vi "Dashboard Main.vi"() -> ()   [LabVIEW 2014]
uses:
  <vilib>/event_ctls.llb/eventvkey.ctl
  <vilib>/Rock Robotics/WPI/Dashboard/WPI_DashboardLogging Global.vi
  <vilib>/Rock Robotics/Network Tables/SD Read Number.vi
  <vilib>/Rock Robotics/Network Tables/SD Read Boolean.vi
  <vilib>/Utility/config.llb/Write Key (String).vi
  <vilib>/Utility/config.llb/Write Key (I32).vi
  <vilib>/Utility/config.llb/NI_LVConfig.lvlib
panel:
  out "Camera Active":bool
  out "Image Message":string="Timeout in Camera Communications"
  out "Camera Image":T1(plugin-control)
  in  "TCP":refnum<k5>
  in  "Rec Mode":enum32{"Stop", "Record", "Playback"}(radio)
  in  "Vision":u16(ring) items=["Camera Off", "USB Camera SW", "USB Camera HW", "IP Camera"]
  in  "Dashboard Tab":T2(tab)
  in  "Camera Settings":T3={"Frame Rate"=30, "Compression"=30, "Size"=1} {"Frame Rate" scale=1.0..30.0; "Size" items=["640x480", "320x240", "160x120"]}
  out "MotorChart R":cluster{"Numeric":dbl, "Numeric":dbl}(graph)
  out "MotorChart L":T4(graph)
  out "MotorSliders R":cluster{"MotorSlide1":dbl, "MotorSlide2":dbl} {"MotorSlide2" scale=-1.0..1.0 scale format="%#_2e"; "MotorSlide1" scale=-1.0..1.0 scale format="%#_2e"}
  out "MotorSliders L":T5 {"MotorSlide4 2" scale=0.0..14.0 scale format="%#_2e"; "MotorSlide2" scale=-1.0..1.0 scale format="%#_2e"; "MotorSlide1" scale=-1.0..1.0 scale format="%#_2e"}
  out "Gyro":dbl(knob) scale=0.0..360.0
  out "JS1 Z":dbl(slide) scale=-1.0..1.0 scale format="%#_2e"
  out "JS1 Graph":cluster{"X":dbl, "Y":dbl}[](graph)
  out "JS1 Buttons":T6
  out "JS2 Z":dbl(slide) scale=-1.0..1.0 scale format="%#_2e"
  out "JS2 Graph":cluster{"X":dbl, "Y":dbl}[](graph)
  out "JS2 Buttons":T6
  out "Mode":T7(ring)=enum."Auto Disabled"
  in  "DB Camera Config":bool
  out "fps":dbl format="%#.1g"
  out "Mbps":dbl format="%#.1g"
  out "Mbps 2":bool
  out "Accel Y":dbl
  out "Accel Z":dbl
  out "Accel X":dbl
  out "LimitSW1":bool
  out "Camera IP":string
  in  "DB/String 9":string
  in  "DB/String 8":string
  in  "DB/String 7":string
  in  "DB/String 6":string
  in  "DB/String 5":string
  in  "DB/String 4":string
  in  "DB/String 3":string
  in  "DB/String 2":string
  in  "DB/String 1":string
  in  "DB/String 0":string
  in  "DB/Slider 0":dbl(slide) scale=0.0..5.0
  in  "DB/Slider 1":dbl(slide) scale=0.0..5.0
  in  "DB/Slider 2":dbl(slide) scale=0.0..5.0
  in  "DB/Slider 3":dbl(slide) scale=0.0..5.0
  out "DB/LED 3":bool
  out "DB/LED 2":bool
  out "DB/LED 1":bool
  out "DB/LED 0":bool
  in  "DB/Button 3":bool
  in  "DB/Button 2":bool
  in  "DB/Button 1":bool
  in  "DB/Button 0":bool caption="New Name"
  in  "Test Slider":dbl(slide) scale=0.0..100.0 scale format="%#_3g"
  in  "On/Off":bool caption="Solenoid"
  in  "Test Name":u16(ring) items=["Select the test to run...", "Example Test", "-------------------------------", "List of tests is built in robot code.", "Replace with your own automated tests."]
  in  "Test Tree":string(tree)
  in  "Motor":cluster{"Value":dbl, "Enable":bool} {"Value" scale=-1.0..1.0 scale format="%#_3g"}
  out "Progress":T8 {"Test Progress" scale=0.0..100.0}
  in  "Rev/Fwd":cluster{"Forward":bool, "Reverse":bool}
  in  "Test Ring":u16(ring) items=["Monochrome", "Color"]
  in  "Listbox":i32(listbox)
  out "Tree":string(tree)
  out "Boolean":bool
  # "Left"
  # "Front"
  # "Right"
  # "Battery"
  # "This tab is a great place for autonomous settings and robot-specific values.\nPlace controls and indicators inside this tab and match name to\nDashboard Variables on robot. You can also delete this comment."
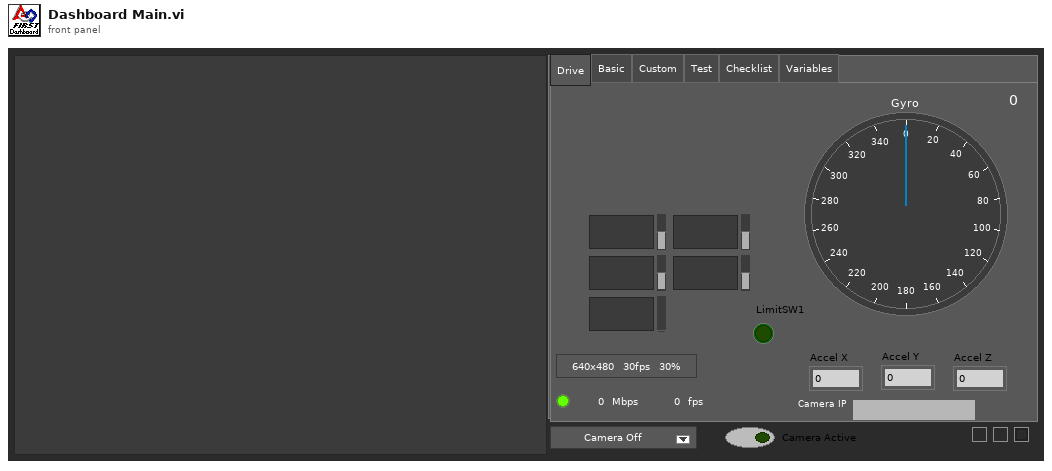
[diagram p1: front panel]
types:
  T1 = typedef "IMAQ Image.ctl" = refnum<image>
  T2 = enum32{"Drive", "Basic", "Custom", "Test", "Checklist", "Variables"}
  T3 = cluster{"Frame Rate":i32, "Compression":i32, "Size":u16}
  T4 = cluster{"Numeric":dbl, "Numeric":dbl, "Battery V":dbl}
  T5 = cluster{"MotorSlide1":dbl, "MotorSlide2":dbl, "MotorSlide4 2":dbl}
  T6 = cluster{bool, bool, bool, bool, bool, bool, bool, bool, bool, bool, bool, bool}
  T7 = enum8{"Tele-Op Disabled", "Tele-Op Enabled", "Auto Disabled", "Auto Enabled", "Test Disabled", "Test Enabled", "Disconnected", "No Code", "E-Stop"}
  T8 = cluster{"Test Progress":u8, "Test Progress Text":string}
  T9 = typedef "Image Type" = u32
  T10 = cluster{"Camera Image":refnum<vi>, "Dashboard Tab":refnum<vi>, "Boolean":refnum<vi>, "Vision":refnum<vi>, "Rec Mode":refnum<vi>, "Test Slider":refnum<vi>, "On/Off ":refnum<vi>, "Test Ring":refnum<vi>, "Rev/Fwd":refnum<vi>, "Test Name":refnum<vi>, "Motor":refnum<vi>, "Progress":refnum<vi>, "CheckList":refnum<vi>, "Tree":refnum<vi>, "Test Tree":refnum<vi>}
  T11 = cluster{"Error Strings":string, "Disable Counts":cluster{u16, u16}, "Rail Faults":cluster{u16, u16, u16}, "Robot IP":string, "DB Mode":u8, "Event Info":cluster{"Name":string, "Type":u8, "Number":u16, "Replay":u8}, "Camera Addr":string}
  T12 = cluster{"Storage":cluster{"Disk Free":u64, "RAM Block":u32, "RAM free":u32}, "CPU Utilization":cluster{"CPU % ISR":sgl, "CPU % Time Crit":sgl, "CPU % Timed Str":sgl, "CPU % High":sgl, "CPU % Above":sgl, "CPU % Normal":sgl, "CPU % Low":sgl}, "CAN":cluster{"% Bus Utilization":sgl, "Bus Off Cnt":u32, "TX_FIFO Full Cnt":u32, "Receive Error Cnt":u8, "Transmit Error Cnt":u8}, "HID":cluster{"HID Outputs":u32, "Rumble Low":u16, "Rumble High":u16}[]}
  T13 = cluster{"Status bits":cluster{"Test Mode":bool, "Autonomous":bool, "Enabled":bool, "Code Start":bool, "Brownout":bool, "Reserved 2":bool, "Reserved 3":bool, "E-Stop":bool}, "Code Trace":cluster{"Disabled":bool, "TeleOp":bool, "Auto":bool, "Test":bool}, "Controller Type":enum16{"unknown", "cRIO", "roboRio"}, "Code?":enum16{"unknown", "noCode", "code"}, "Battery V":dbl}
  T14 = cluster{"Control Bits":cluster{"TestMode":bool, "Autonomous":bool, "Enabled":bool, "FMS Present":bool, bool, bool, bool, "E-Stop":bool}, "Team Station ":u8, "Countdown":sgl, "Joystick Values":cluster{"Axes":dbl[], "Buttons":bool[], "POVs":i16[]}[]}
  T15 = cluster{"Axes":dbl[], "Buttons":bool[], "POVs":i16[]}[]
  T16 = cluster{"Axes":dbl[], "Buttons":bool[], "POVs":i16[]}
  T17 = cluster{"Buttons[0]":bool, "Buttons[1]":bool, "Buttons[2]":bool, "Buttons[3]":bool, "Buttons[4]":bool, "Buttons[5]":bool, "Buttons[6]":bool, "Buttons[7]":bool, "Buttons[8]":bool, "Buttons[9]":bool, "Buttons[10]":bool, "Buttons[11]":bool}
  T18 = typedef "NI_LVConfig.lvlib/Config Data RefNum.ctl" = refnum<k1>
  T19 = cluster{"Operation":enum16{"Update", "Clear"}, "Color Box":u32}[]
  T20 = typedef "eventvkey.ctl" = enum16{"ASCII", "Enter", "Return", "Shift", "Ctrl", "Alt", "Cmd", "Opt", "Caps", "NumLock", "Clear", "Break", "Up", "Down", "Left", "Right", "Insert", "Delete", "Home", "End", "PageUp", "PageDown", "Escape", "Help", "Pause", "ScrollLock", "F1", "F2", "F3", "F4", "F5", "F6", "F7", "F8", "F9", "F10", "F11", "F12", "F13", "F14", "F15", "F16", "F17", "F18", "F19", "F20", "F21", "F22", "F23", "F24", "Play", "VolumeUp", "VolumeDown", "Mute", "Two Byte Char"}
  T21 = cluster{"Image Size":bool, "Image Type":bool, "Pixel Value":bool, "ROI Information":bool, "Zoom Factor":bool}
  T22 = enum8{"Enabled", "Disabled", "Disabled and Grayed Out"}
  T23 = cluster{"Operation":enum16{"Update", "Clear"}, "Color Box":u32}
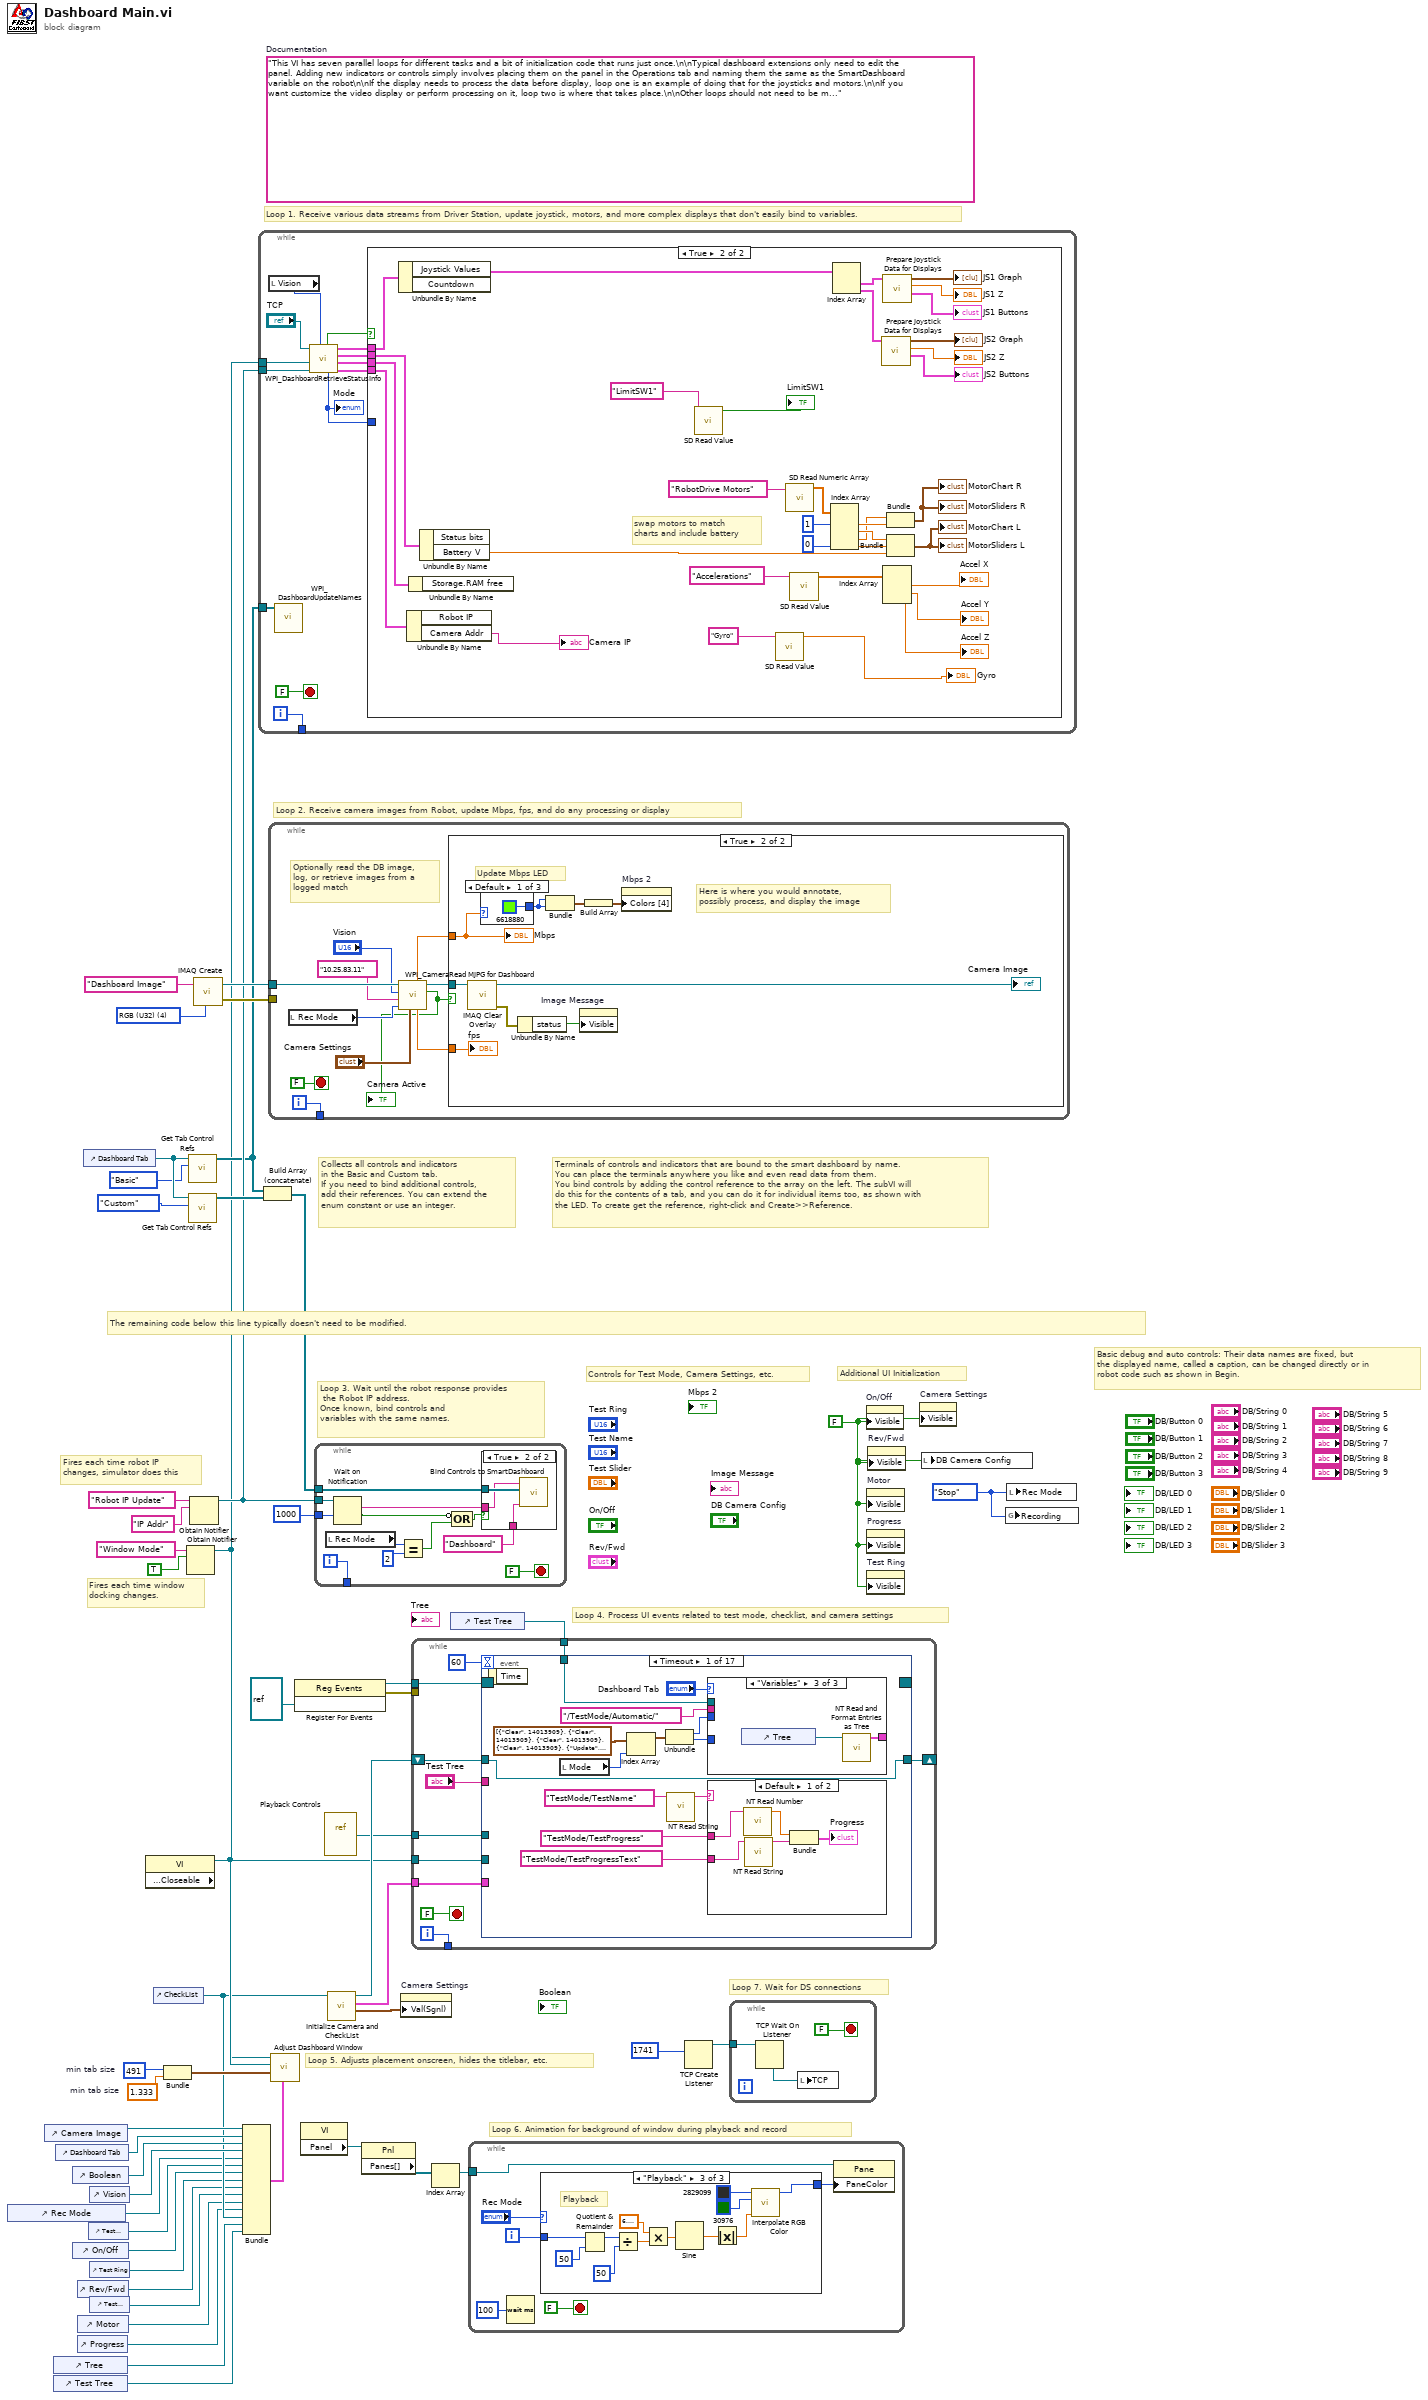
[diagram p0: block diagram]
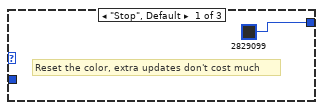
[diagram p3: hidden frame]
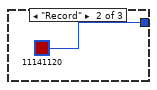
[diagram p4: hidden frame]
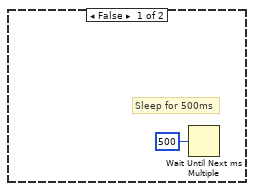
[diagram p6: hidden frame]
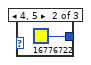
[diagram p7: hidden frame]
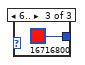
[diagram p8: hidden frame]
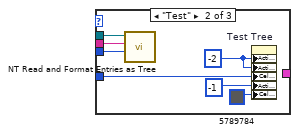
[diagram p10: hidden frame]
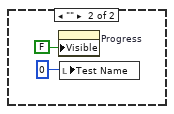
[diagram p11: hidden frame]
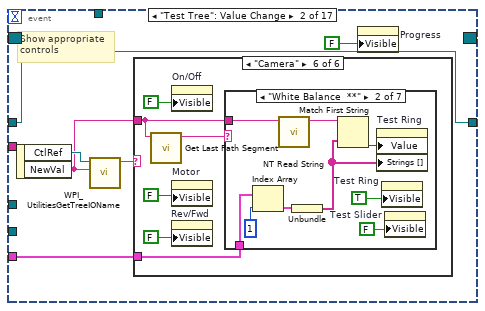
[diagram p12: hidden frame]
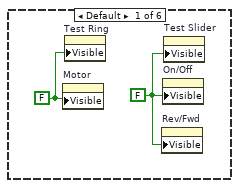
[diagram p13: hidden frame]
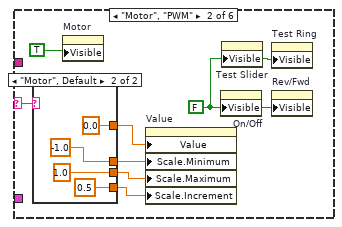
[diagram p14: hidden frame]
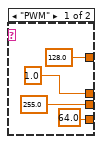
[diagram p15: hidden frame]
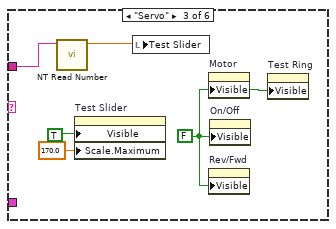
[diagram p16: hidden frame]
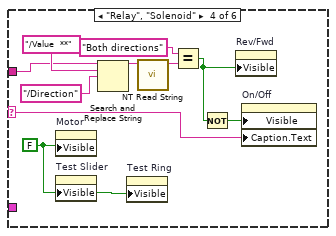
[diagram p17: hidden frame]
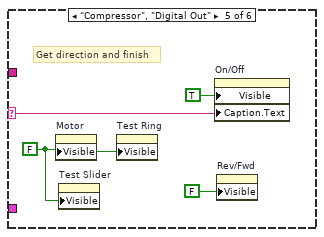
[diagram p18: hidden frame]
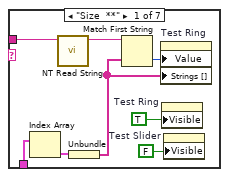
[diagram p19: hidden frame]
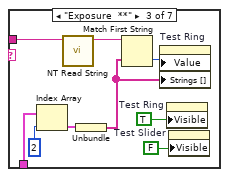
[diagram p20: hidden frame]
diagram:
  w24 = 491  # min tab size
  w23 = 1.333  # min tab size
  w32 = enum32{"Stop", "Record", "Playback"}."Stop" ("Rec Mode")
  w6 = FALSE ("Visible")
  (unwired) "This VI has seven parallel loops for different tasks and a bit of initialization code that runs just once.\n\nTypical dashboard extensions only need to edit the panel. Adding new indicators or controls simply involves placing them on the panel in the Operations tab and naming them the same as the SmartDashboard variable on the robot\n\nIf the display needs to process the data before display, loop one is an example of doing that for the joysticks and motors.\n\nIf you want customize the video display or perform processing on it, loop two is where that takes place.\n\nOther loops should not need to be modified. They are pretty standard, and document the task they perform."  # Documentation
  w52 = T9 4 items=["Grayscale (U8)", "Grayscale (I16)", "Grayscale (SGL)", "Complex (CSG)", "RGB (U32)", "HSL (U32)", "RGB (U64)"] ("Image Type")
  # "Loop 7. Wait for DS connections"
  # "Basic debug and auto controls: Their data names are fixed, but\nthe displayed name, called a caption, can be changed directly or in\nrobot code such as shown in Begin."
  # "Controls for Test Mode, Camera Settings, etc."
  # "Additional UI Initialization"
  # "Loop 6. Animation for background of window during playback and record"
  # "Fires each time robot IP\nchanges, simulator does this"
  # "Fires each time window\ndocking changes."
  # "Collects all controls and indicators\nin the Basic and Custom tab.\nIf you need to bind additional controls,\nadd their references. You can extend the\nenum constant or use an integer."
  # "The remaining code below this line typically doesn't need to be modified."
  # "Loop 4. Process UI events related to test mode, checklist, and camera settings"
  # "Terminals of controls and indicators that are bound to the smart dashboard by name.\nYou can place the terminals anywhere you like and even read data from them.\nYou bind controls by adding the control reference to the array on the left. The subVI will\ndo this for the contents of a tab, and you can do it for individual items too, as shown with\nthe LED. To create get the reference, right-click and Create>>Reference."
  # "Loop 3. Wait until the robot response provides\n the Robot IP address.\nOnce known, bind controls and\nvariables with the same names."
  # "Loop 5. Adjusts placement onscreen, hides the titlebar, etc."
  # "Loop 1. Receive various data streams from Driver Station, update joystick, motors, and more complex displays that don't easily bind to variables."
  # "Loop 2. Receive camera images from Robot, update Mbps, fps, and do any processing or display"
  n1 = control-ref of="Rec Mode"() -> (w12:refnum<vi>)
  n2 = control-ref of="Camera Image"() -> (w27:refnum<vi>)
  n3 = control-ref of="Tree"() -> (w16:refnum<vi>)
  n4 = control-ref of="Test Tree"() -> (w15:refnum<vi>)
  n5 = control-ref of="Dashboard Tab"() -> (w26:refnum<vi>)
  n6 = control-ref of="Boolean"() -> (w21:refnum<vi>)
  n7 = control-ref of="On/Off"() -> (w10:refnum<vi>)
  n8 = control-ref of="Progress"() -> (w7:refnum<vi>)
  n9 = control-ref of="Rev/Fwd"() -> (w8:refnum<vi>)
  n10 = control-ref of="Motor"() -> (w13:refnum<vi>)
  n11 = control-ref of="Dashboard Tab"() -> (w30:refnum<vi>)
  n12 = control-ref of="Test Slider"() -> (w11:refnum<vi>)
  n13 = control-ref of="Vision"() -> (w25:refnum<vi>)
  n14 = control-ref of="Test Ring"() -> (w9:refnum<vi>)
  n15 = control-ref of="Test Name"() -> (w14:refnum<vi>)
  n16 = property class="VI" props=["Front Panel.Closeable"]() -> (reference out=w31:refnum<vi>)  [unwired: 2 in, 2 out]
  n17 = control-ref of="CheckList"() -> (w17:refnum<vi>)
  n18 = Bundle("min tab size"=w24, "min tab size"=w23) -> (w22:cluster{"min tab size":i32, "min tab size":dbl})  [unwired: 1 in]
  n19 = Obtain Notifier(name (unnamed)="Window Mode", notification data type=TRUE) -> (notifier out=w3:refnum<notifier>)  [unwired: 2 in, 2 out]
  n20 = call <vilib>:"Get Tab Control Refs.vi"("Page Index"=T2."Basic" ("Dashboard Tab"), "TabControl in"=w30) -> ("ControlsOnPage"=w4:refnum<vi>[])  [unwired: 9 in]
  n21 = call <vilib>:"Get Tab Control Refs.vi"("Page Index"=T2."Custom" ("Dashboard Tab"), "TabControl in"=w30) -> ("ControlsOnPage"=w29:refnum<vi>[])  [unwired: 9 in]
  n22 = Obtain Notifier(name (unnamed)="Robot IP Update", notification data type="IP Addr" ("name (unnamed)")) -> (notifier out=w5:refnum<notifier>)  [unwired: 2 in, 2 out]
  n23 = call "IMAQ Create"("Image Name"="Dashboard Image", "Image Type"=w52) -> ("New Image"=w50:T1, "error out"=w49:errorcluster)  [unwired: 2 in, 1 out]
  n24 = Bundle("Camera Image"=w27, "Dashboard Tab"=w26, "Boolean"=w21, "Vision"=w25, "Rec Mode"=w12, "Test Slider"=w11, "On/Off"=w10, "Test Ring"=w9, "Rev/Fwd"=w8, "Test Name"=w14, "Motor"=w13, "Progress"=w7, "CheckList"=w17, "Tree"=w16, "Test Tree"=w15) -> (w18:T10)  [unwired: 1 in]
  n25 = while {
    tunnel: [w64] -> _
    tunnel: w5 -> [w58]
    tunnel: w4 -> [w57]
    tunnel: w3 -> [w53]
    i -> [w64]
    stop <- FALSE stop-if-true
    n26 = local read "Vision"() -> (w55:u16)
    n27 = call <vilib>:"WPI_DashboardUpdateNames.vi"("Controls on Tab"=w57) -> ()  [unwired: 11 in]
    n28 = call <vilib>:"WPI_DashboardRetrieveStatusInfo.vi"("Vision"=w55, "Binding Refnum"=w58, "Window Mode Notifier"=w53, "TCP Cnx"="TCP") -> ("Power and Errors"=w59:T11, "Robot Metrics"=w62:T12, "Status Info"=w63:T13, "Control Info"=w60:T14, "Robot Mode"=w56:T7, "Process?"=w61:bool)  [unwired: 2 in]
    "Mode" <- w56
    n29 = case shown="True" w61 {
      tunnel: w63 -> [_ w99]
      tunnel: w62 -> [_ w98]
      tunnel: w60 -> [_ w97]
      tunnel: w59 -> [_ w96]
      tunnel: w56 -> [_ _]
      frame False {
      }
      frame True {
        # "swap motors to match\ncharts and include battery"
        n30 = Unbundle By Name(w97) -> ("Joystick Values"=w84:T15)  [unwired: 1 out]
        n31 = Unbundle By Name(w96) -> ("Camera Addr"=→"Camera IP":string)  [unwired: 1 out]
        n32 = Unbundle By Name(w98) -> ()  [unwired: 1 out]
        n33 = Unbundle By Name(w99) -> ("Battery V"=w85:dbl)  [unwired: 1 out]
        n34 = call-poly <vilib>:"SD Read Value.vi"("Name"="LimitSW1") -> ("Boolean"=→"LimitSW1":bool)  [unwired: 8 in, 2 out]
        n35 = call-poly <vilib>:"SD Read Value.vi"("Name"="Gyro") -> ("Numeric"=→"Gyro":dbl)  [unwired: 8 in, 2 out]
        n36 = call <vilib>:"SD Read Numeric Array.vi"("Name"="RobotDrive Motors") -> ("Numeric Array"=w87:dbl[])  [unwired: 8 in, 2 out]
        n37 = call-poly <vilib>:"SD Read Value.vi"("Name"="Accelerations") -> ("Numeric Array"=w73:dbl[])  [unwired: 8 in, 2 out]
        n38 = Index Array(array=w87, index #1=1, index #4=0) -> (element #1=w91:dbl, element #2=w92:dbl, element #3=w90:dbl, element #4=w95:dbl)  [unwired: 2 in]
        n39 = Index Array(array=w84) -> (element #1=w83:T16, element #2=w78:T16)  [unwired: 2 in]
        n40 = call "Prepare Joystick Data for Displays.vi"("Joystick Values"=w78) -> ("Buttons"=→"JS2 Buttons":T17, "Z Axis"=→"JS2 Z":dbl, "Cartesian Data"=→"JS2 Graph":cluster{"X axis":dbl, "X axis":dbl}[])  [unwired: 8 in]
        n41 = call "Prepare Joystick Data for Displays.vi"("Joystick Values"=w83) -> ("Buttons"=→"JS1 Buttons":T17, "Z Axis"=→"JS1 Z":dbl, "Cartesian Data"=→"JS1 Graph":cluster{"X axis":dbl, "X axis":dbl}[])  [unwired: 8 in]
        n42 = Index Array(array=w73) -> (element #1=→"Accel X":dbl, element #2=→"Accel Y":dbl, element #3=→"Accel Z":dbl)  [unwired: 3 in]
        n43 = Bundle("Numeric"=w90, "Numeric"=w91) -> (→"MotorChart R" →"MotorSliders R":cluster{"Numeric":dbl, "Numeric":dbl})  [unwired: 1 in]
        n44 = Bundle("Numeric"=w92, "Numeric"=w95, "Battery V"=w85) -> (→"MotorChart L" →"MotorSliders L":T4)  [unwired: 1 in]
      }
    }
  }
  n45 = Build Array (concatenate)(w4, w29) -> (w28:refnum<vi>[])
  n46 = while {
    tunnel: w50 -> [w108]
    tunnel: w49 -> [_]
    tunnel: [w109] -> _
    i -> [w109]
    stop <- FALSE stop-if-true
    # "Optionally read the DB image,\nlog, or retrieve images from a\nlogged match"
    n47 = local read "Rec Mode"() -> (w103:enum32{"Stop", "Record", "Playback"})
    n48 = call <vilib>:"WPI_CameraRead MJPG for Dashboard.vi"("Camera Settings"="Camera Settings", "Rec Mode"=w103, "Camera IP"="10.25.83.11", "Camera Mode"="Vision", "Refnum in"=w108) -> ("Active"=w101:bool, "Refnum out"=w107:T1, "FPS"=w106:dbl, "Bandwidth (Mbps)"=w105:dbl)  [unwired: 3 in]
    "Camera Active" <- w101
    n49 = case shown="True" w101 {
      tunnel: w107 -> [_ w115]
      tunnel: w105 -> [_ w114]
      tunnel: w106 -> [_ w112]
      frame False {
        # "Sleep for 500ms"
        n50 = Wait Until Next ms Multiple(millisecond multiple=u32 500) -> ()  [unwired: 1 out]
      }
      frame True {
        # "Here is where you would annotate,\npossibly process, and display the image"
        # "Update Mbps LED"
        n51 = call "IMAQ Clear Overlay"("Image"=w115) -> ("error out"=w119:errorcluster, "Image Out"=→"Camera Image":T1)  [unwired: 2 in, 7 out]
        n52 = case shown="Default" w114 {
          tunnel: [u32 6618880 ("Color Box") u32 16776722 ("Color Box") u32 16716800 ("Color Box")] -> w116
          frame Default {
          }
          frame 4, 5 {
          }
          frame 6.. {
          }
        }
        n53 = Unbundle By Name(w119) -> ("status"=w120:bool)
        n54 = Bundle("Color Box"=w116, "Color Box"=w116) -> (w118:cluster{"Color Box":u32, "Color Box":u32})  [unwired: 1 out]
        n55 = property on="Image Message" class="Str"("Visible"=w120) -> ()  [unwired: 2 in, 2 out]
        n56 = Build Array(w118) -> (w117:cluster{"Color Box":u32, "Color Box":u32}[])
        n57 = property on="Mbps 2" class="Bool (strict)"("Colors [4]"=w117) -> ()  [unwired: 2 in, 2 out]
        "Mbps" <- w114
        "fps" <- w112
      }
    }
  }
  n58 = call "Adjust Dashboard Window.vi"("Sizing Refnums"=w18, "Size Constraints"=w22, "VI"=w31, "Notifier in"=w3) -> ()  [unwired: 8 in]
  n59 = register-events(refnum<vi> refnum) -> (reference out=w36:refnum<event-registration>, error out=w35:errorcluster)  [unwired: 2 in]
  n60 = property class="VI"() -> ("Panel"=w39:refnum<vi>)  [unwired: 2 in, 2 out]
  n61 = while {
    tunnel: w28 -> [w135]
    tunnel: w5 -> [w133]
    tunnel: [w131] -> _
    tunnel: u32 1000 ("milliseconds to wait") -> [w130]
    i -> [w131]
    stop <- FALSE stop-if-true
    n62 = local read "Rec Mode"() -> (w126:enum32{"Stop", "Record", "Playback"})
    n63 = Wait on Notification(notifier=w133, timeout in ms (-1)=w130) -> (notification=w132:string, timed out?=w128:bool)  [unwired: 2 in, 2 out]
    n64 = Equal?(x=w126, y=u16 2 ("Rec Mode")) -> (x = y?=w127:bool)
    n65 = Compound Arithmetic op=OR(invert w128, w127) -> (w129:bool)
    n66 = case shown="True" w129 {
      tunnel: w135 -> [_ w138]
      tunnel: w132 -> [_ w137]
      tunnel: "Dashboard" -> [_ w136]
      frame False {
      }
      frame True {
        n67 = call <vilib>:"Bind Controls to SmartDashboard.vi"("Client Name"=w136, "Bound Control Refs"=w138, "Server IP Address"=w137) -> ()  [unwired: 9 in]
      }
    }
  }
  n68 = vi-ref "Playback Controls.vi"() -> (w37:refnum<vi>)
  n69 = call "Initialize Camera and CheckList.vi"("ListBox in"=w17) -> ("Cluster"=w43:cluster{"value":i32, "value":i32, "index":i32}, "Array"=w44:cluster{string[]}[], "File Refnum"=w42:T18)  [unwired: 8 in]
  n70 = property class="Pnl"(reference=w39) -> ("Panes[]"=w40:refnum<vi>[])  [unwired: 1 in, 2 out]
  n71 = property on="Camera Settings" class="Clust (strict)"("Val(Sgnl)"=w43) -> ()  [unwired: 2 in, 2 out]
  n72 = Index Array(array=w40) -> (element=w38:refnum<vi>)  [unwired: 1 in]
  n73 = control-ref of="Test Tree"() -> (w41:refnum<vi>)
  n74 = while {
    tunnel: w44 -> [w146]
    shift-right: [w145] -> _
    shift-left: w42 -> [w144]
    tunnel: [w143] -> _
    tunnel: w41 -> [w142]
    tunnel: w37 -> [w141]
    tunnel: w36 -> [w140]
    tunnel: w35 -> [_]
    tunnel: w31 -> [w139]
    i -> [w143]
    stop <- FALSE stop-if-true
    n75 = event shown="[0] Timeout" {
      selector: w140 -> [_ _ _ _ _ _ _ _ _ _ _ _ _ _ _ _ _]
      dyn-events: [_ _ _ _ _ _ _ _ _ _ _ _ _ w384 _ _ _] -> _
      timeout: u32 60 ("milliseconds to wait") -> [_ _ _ _ _ _ _ _ _ _ _ _ _ _ _ _ _]
      tunnel: w142 -> [w158 _ _ _ _ _ _ _ _ _ _ _ _ _ _ _ _]
      tunnel: "Test Tree" -> [_ _ _ _ _ _ _ _ w353 w361 w363 w367 w375 _ _ _ _]
      tunnel: w146 -> [_ w180 _ _ _ _ w317 w347 _ _ _ _ _ _ _ _ _]
      tunnel: [w154 w179 w278 w283 w291 w303 w316 w340 w352 w359 w362 w366 w374 w386 w400 w401 w411] -> w145
      tunnel: w144 -> [w154 w179 w278 w283 w291 w303 w315 w340 w352 w359 w362 w366 w374 w386 w400 w401 w411]
      tunnel: w141 -> [_ _ _ _ _ _ _ _ _ _ _ _ _ w387 _ w404 _]
      tunnel: w139 -> [_ _ _ _ _ _ _ _ _ _ _ _ _ w382 _ _ _]
      event Timeout {
        n76 = event-data() -> ()  [unwired: 1 in, 1 out]
        n77 = local read "Mode"() -> (w157:T7)
        n78 = Index Array(array=T19 [{"Operation"=enum."Clear", "Color Box"=14013909}, {"Operation"=enum."Clear", "Color Box"=14013909}, {"Operation"=enum."Clear", "Color Box"=14013909}, {"Operation"=enum."Clear", "Color Box"=14013909}, {"Operation"=enum."Update", "Color Box"=14013909}, {"Operation"=enum."Update", "Color Box"=16777215}, {"Operation"=enum."Clear", "Color Box"=14013909}, {"Operation"=enum."Clear", "Color Box"=14013909}, {"Operation"=enum."Clear", "Color Box"=14013909}], index=w157) -> (element=w152:T23)
        n79 = Unbundle(w152) -> ("Operation"=w151:enum16{"Update", "Clear"}, "Color Box"=w150:u32)
        n80 = call <vilib>:"NT Read String.vi"("Name"="TestMode/TestName") -> ("String"=w161:string)  [unwired: 9 in, 1 out]
        n81 = case shown="\"Variables\"" "Dashboard Tab" {
          tunnel: w158 -> [_ w169 _]
          tunnel: "/TestMode/Automatic/" ("Name Pattern") -> [_ w168 _]
          tunnel: w151 -> [_ w167 _]
          tunnel: [_ _ w171] -> _
          tunnel: w150 -> [_ w163 _]
          frame "Custom", Default {
          }
          frame "Test" {
            w166 = -2 ("Active Item:Row Number")
            n82 = call <vilib>:"NT Read and Format Entries as Tree.vi"("Operation"=w167, "Name Pattern"=w168, "Tree Refnum"=w169) -> ()  [unwired: 7 in, 2 out]
            n83 = property on="Test Tree" class="Tree (strict)"("Active Item Row Number"=w166, "ActiveColNum"=w166, "CellBG"=w163, "Active Item Row Number"=-1 ("Active Item:Row Number"), "CellBG"=u32 5789784 ("Color Box")) -> ()  [unwired: 2 in, 2 out]
          }
          frame "Variables" {
            n84 = control-ref of="Tree"() -> (w170:refnum<vi>)
            n85 = call <vilib>:"NT Read and Format Entries as Tree.vi"("Tree Refnum"=w170) -> ("Formatted Strings"=w171:cluster{"Name":string, "Value":string}[])  [unwired: 9 in, 1 out]
          }
        }
        n86 = case shown="Default" w161 {
          tunnel: "TestMode/TestProgress" ("Name") -> [w173 _]
          tunnel: "TestMode/TestProgressText" ("Name") -> [w172 _]
          frame Default {
            n87 = call <vilib>:"NT Read Number.vi"("Name"=w173) -> ("Numeric"=w174:dbl)  [unwired: 9 in, 1 out]
            n88 = call <vilib>:"NT Read String.vi"("Name"=w172) -> ("String"=w175:string)  [unwired: 9 in, 1 out]
            n89 = Bundle("Numeric"=w174, "String"=w175) -> (→"Progress":cluster{"Numeric":dbl, "String":string})  [unwired: 1 in]
          }
          frame "" {
            n90 = property on="Progress" class="Clust (strict)"("Visible"=FALSE) -> ()  [unwired: 2 in, 2 out]
            n91 = local write "Test Name"(u16 0) -> ()
          }
        }
      }
      event "Test Tree": Value Change {
        # "Show appropriate\ncontrols"
        n92 = event-data() -> ("CtlRef"=w183:refnum<vi>, "NewVal"=w181:string)  [unwired: 1 in]
        n93 = call <vilib>:"WPI_UtilitiesGetTreeIOName.vi"("NewVal"=w181, "TreeControl in"=w183) -> ("I/O Name"=w184:string)  [unwired: 9 in]
        n94 = case shown="\"Camera\"" w184 {
          selector: w184 -> [_ w191 _ w209 w218 _]
          tunnel: w181 -> [_ _ w206 w208 _ w225]
          tunnel: w180 -> [_ _ _ _ _ w224]
          frame Default {
            w186 = FALSE ("Visible")
            w185 = FALSE ("Visible")
            n95 = property on="Motor" class="Clust (strict)"("Visible"=w185) -> ()  [unwired: 2 in, 2 out]
            n96 = property on="Test Ring" class="Ring (strict)"("Visible"=w185) -> ()  [unwired: 2 in, 2 out]
            n97 = property on="Rev/Fwd" class="Clust (strict)"("Visible"=w186) -> ()  [unwired: 2 in, 2 out]
            n98 = property on="On/Off" class="Bool (strict)"("Visible"=w186) -> ()  [unwired: 2 in, 2 out]
            n99 = property on="Test Slider" class="Slide (strict)"("Visible"=w186) -> ()  [unwired: 2 in, 2 out]
          }
          frame "Motor", "PWM" {
            w192 = FALSE ("Visible")
            n100 = case shown="\"Motor\", Default" w191 {
              tunnel: [1.0 ("Value") -1.0 ("Value")] -> w190
              tunnel: [255.0 ("Value") 1.0 ("Value")] -> w189
              tunnel: [128.0 ("Value") 0.0 ("Value")] -> w188
              tunnel: [64.0 ("Value") 0.5 ("Value")] -> w187
              frame "PWM" {
              }
              frame "Motor", Default {
              }
            }
            n101 = property on="Motor" class="Clust (strict)"("Visible"=TRUE) -> ()  [unwired: 2 in, 2 out]
            n102 = property on="Value" class="Slide (strict)"("Value"=w188, "Scale.Minimum"=w190, "Scale.Maximum"=w189, "Scale.Increment"=w187) -> ()  [unwired: 2 in, 2 out]
            n103 = property on="On/Off" class="Bool (strict)"("Visible"=w192) -> ()  [unwired: 2 in, 2 out]
            n104 = property on="Test Slider" class="Slide (strict)"("Visible"=w192) -> ()  [unwired: 2 in, 2 out]
            n105 = property on="Test Ring" class="Ring (strict)"("Visible"=w192) -> ()  [unwired: 2 in, 2 out]
            n106 = property on="Rev/Fwd" class="Clust (strict)"("Visible"=w192) -> ()  [unwired: 2 in, 2 out]
          }
          frame "Servo" {
            w204 = FALSE ("Visible")
            n107 = call <vilib>:"NT Read Number.vi"("Name"=w206) -> ("Numeric"=w205:dbl)  [unwired: 9 in, 1 out]
            n108 = property on="Test Slider" class="Slide (strict)"("Visible"=TRUE, "Scale.Maximum"=170.0 ("Scale.Range:Maximum")) -> ()  [unwired: 2 in, 2 out]
            n109 = local write "Test Slider"(w205) -> ()
            n110 = property on="Motor" class="Clust (strict)"("Visible"=w204) -> ()  [unwired: 2 in, 2 out]
            n111 = property on="Rev/Fwd" class="Clust (strict)"("Visible"=w204) -> ()  [unwired: 2 in, 2 out]
            n112 = property on="On/Off" class="Bool (strict)"("Visible"=w204) -> ()  [unwired: 2 in, 2 out]
            n113 = property on="Test Ring" class="Ring (strict)"("Visible"=w204) -> ()  [unwired: 2 in, 2 out]
          }
          frame "Relay", "Solenoid" {
            w207 = FALSE ("Visible")
            n114 = property on="Motor" class="Clust (strict)"("Visible"=w207) -> ()  [unwired: 2 in, 2 out]
            n115 = property on="Test Slider" class="Slide (strict)"("Visible"=w207) -> ()  [unwired: 2 in, 2 out]
            n116 = Search and Replace String(input string=w208, search string="/Value  **", replace string="/Direction") -> (result string=w214:string)  [unwired: 5 in, 3 out]
            n117 = property on="Test Ring" class="Ring (strict)"("Visible"=w207) -> ()  [unwired: 2 in, 2 out]
            n118 = call <vilib>:"NT Read String.vi"("Name"=w214) -> ("String"=w212:string)  [unwired: 9 in, 1 out]
            n119 = Equal?(x="Both directions", y=w212) -> (x = y?=w210:bool)
            n120 = Not(x=w210) -> (.not. x?=w211:bool)
            n121 = property on="Rev/Fwd" class="Clust (strict)"("Visible"=w210) -> ()  [unwired: 2 in, 2 out]
            n122 = property on="On/Off" class="Bool (strict)"("Visible"=w211, "Caption.Text"=w209) -> ()  [unwired: 2 in, 2 out]
          }
          frame "Compressor", "Digital Out" {
            w217 = FALSE ("Visible")
            # "Get direction and finish"
            n123 = property on="Motor" class="Clust (strict)"("Visible"=w217) -> ()  [unwired: 2 in, 2 out]
            n124 = property on="Test Slider" class="Slide (strict)"("Visible"=w217) -> ()  [unwired: 2 in, 2 out]
            n125 = property on="Test Ring" class="Ring (strict)"("Visible"=w217) -> ()  [unwired: 2 in, 2 out]
            n126 = property on="On/Off" class="Bool (strict)"("Visible"=TRUE, "Caption.Text"=w218) -> ()  [unwired: 2 in, 2 out]
            n127 = property on="Rev/Fwd" class="Clust (strict)"("Visible"=FALSE) -> ()  [unwired: 2 in, 2 out]
          }
          frame "Camera" {
            n128 = call <vilib>:"Get Last Path Segment.vi"("String in"=w225) -> ("String out"=w226:string)  [unwired: 10 in]
            n129 = property on="On/Off" class="Bool (strict)"("Visible"=FALSE) -> ()  [unwired: 2 in, 2 out]
            n130 = property on="Motor" class="Clust (strict)"("Visible"=FALSE) -> ()  [unwired: 2 in, 2 out]
            n131 = property on="Rev/Fwd" class="Clust (strict)"("Visible"=FALSE) -> ()  [unwired: 2 in, 2 out]
            n132 = case shown="\"White Balance  **\"" w226 {
              tunnel: w225 -> [w232 w241 w250 w259 w268 _ w274]
              tunnel: w224 -> [w230 w238 w247 w256 w265 _ _]
              frame "Size  **" {
                n133 = Index Array(array=w230) -> (element=w229:cluster{string[]})  [unwired: 1 in]
                n134 = call <vilib>:"NT Read String.vi"("Name"=w232) -> ("String"=w231:string)  [unwired: 9 in, 1 out]
                n135 = Unbundle(w229) -> (w227:string[])
                n136 = Match First String(2:w227, 3:w231) -> (0:w228:i32)  [unwired: 1 out]
                n137 = property on="Test Ring" class="Ring (strict)"("Value"=w228, "Strings []"=w227) -> ()  [unwired: 2 in, 2 out]
                n138 = property on="Test Ring" class="Ring (strict)"("Visible"=TRUE) -> ()  [unwired: 2 in, 2 out]
                n139 = property on="Test Slider" class="Slide (strict)"("Visible"=FALSE) -> ()  [unwired: 2 in, 2 out]
              }
              frame "White Balance  **" {
                n140 = Index Array(array=w238, index=1) -> (element=w239:cluster{string[]})
                n141 = call <vilib>:"NT Read String.vi"("Name"=w241) -> ("String"=w240:string)  [unwired: 9 in, 1 out]
                n142 = Unbundle(w239) -> (w236:string[])
                n143 = Match First String(2:w236, 3:w240) -> (0:w235:i32)  [unwired: 1 out]
                n144 = property on="Test Ring" class="Ring (strict)"("Value"=w235, "Strings []"=w236) -> ()  [unwired: 2 in, 2 out]
                n145 = property on="Test Ring" class="Ring (strict)"("Visible"=TRUE) -> ()  [unwired: 2 in, 2 out]
                n146 = property on="Test Slider" class="Slide (strict)"("Visible"=FALSE) -> ()  [unwired: 2 in, 2 out]
              }
              frame "Exposure  **" {
                n147 = Index Array(array=w247, index=2) -> (element=w248:cluster{string[]})
                n148 = call <vilib>:"NT Read String.vi"("Name"=w250) -> ("String"=w249:string)  [unwired: 9 in, 1 out]
                n149 = Unbundle(w248) -> (w244:string[])
                n150 = Match First String(2:w244, 3:w249) -> (0:w245:i32)  [unwired: 1 out]
                n151 = property on="Test Ring" class="Ring (strict)"("Value"=w245, "Strings []"=w244) -> ()  [unwired: 2 in, 2 out]
                n152 = property on="Test Ring" class="Ring (strict)"("Visible"=TRUE) -> ()  [unwired: 2 in, 2 out]
                n153 = property on="Test Slider" class="Slide (strict)"("Visible"=FALSE) -> ()  [unwired: 2 in, 2 out]
              }
              frame "Exposure Priority  **" {
                n154 = Index Array(array=w256, index=3) -> (element=w257:cluster{string[]})
                n155 = call <vilib>:"NT Read String.vi"("Name"=w259) -> ("String"=w258:string)  [unwired: 9 in, 1 out]
                n156 = Unbundle(w257) -> (w253:string[])
                n157 = Match First String(2:w253, 3:w258) -> (0:w254:i32)  [unwired: 1 out]
                n158 = property on="Test Ring" class="Ring (strict)"("Value"=w254, "Strings []"=w253) -> ()  [unwired: 2 in, 2 out]
                n159 = property on="Test Ring" class="Ring (strict)"("Visible"=TRUE) -> ()  [unwired: 2 in, 2 out]
                n160 = property on="Test Slider" class="Slide (strict)"("Visible"=FALSE) -> ()  [unwired: 2 in, 2 out]
              }
              frame "Color Enable  **" {
                n161 = Index Array(array=w265, index=4) -> (element=w266:cluster{string[]})
                n162 = call <vilib>:"NT Read String.vi"("Name"=w268) -> ("String"=w267:string)  [unwired: 9 in, 1 out]
                n163 = Unbundle(w266) -> (w262:string[])
                n164 = Match First String(2:w262, 3:w267) -> (0:w263:i32)  [unwired: 1 out]
                n165 = property on="Test Ring" class="Ring (strict)"("Value"=w263, "Strings []"=w262) -> ()  [unwired: 2 in, 2 out]
                n166 = property on="Test Ring" class="Ring (strict)"("Visible"=TRUE) -> ()  [unwired: 2 in, 2 out]
                n167 = property on="Test Slider" class="Slide (strict)"("Visible"=FALSE) -> ()  [unwired: 2 in, 2 out]
              }
              frame Default {
                n168 = property on="Test Ring" class="Ring (strict)"("Visible"=FALSE) -> ()  [unwired: 2 in, 2 out]
                n169 = property on="Test Slider" class="Slide (strict)"("Visible"=FALSE) -> ()  [unwired: 2 in, 2 out]
              }
              frame "Brightness  **", "Color Level  **", "Compression  **", "FPS  **", "Sharpness  **" {
                n170 = call <vilib>:"NT Read Number.vi"("Name"=w274) -> ("Numeric"=w273:dbl)  [unwired: 9 in, 1 out]
                n171 = local write "Test Slider"(w273) -> ()
                n172 = property on="Test Slider" class="Slide (strict)"("Visible"=TRUE, "Scale.Maximum"=100.0 ("Scale.Range:Maximum")) -> ()  [unwired: 2 in, 2 out]
                n173 = property on="Test Ring" class="Ring (strict)"("Visible"=FALSE) -> ()  [unwired: 2 in, 2 out]
              }
            }
          }
        }
        n174 = property on="Progress" class="Clust (strict)"("Visible"=FALSE) -> ()  [unwired: 2 in, 2 out]
      }
      event "Test Name": Mouse Enter {
        # "Populate the ring with the list of tests"
        n175 = event-data() -> ()  [unwired: 1 in, 1 out]
        n176 = call <vilib>:"NT Read String Array.vi"("Name"="TestMode/TestList") -> ("String Array"=w282:string[])  [unwired: 9 in, 1 out]
        n177 = Build Array (concatenate)("Select the test to run...", w282) -> (w281:string[])
        n178 = property on="Test Name" class="Ring (strict)"("Strings []"=w281) -> ()  [unwired: 2 in, 2 out]
      }
      event "Test Name": Value Change {
        w284 = FALSE ("Visible")
        # "Tell the robot the test name to run"
        n179 = event-data() -> ("NewVal"=w288:u16)  [unwired: 1 in]
        n180 = property on="Test Name" class="Ring (strict)"() -> ("Strings []"=w289:string[])  [unwired: 2 in, 2 out]
        n181 = local write "Progress"(T8 {"Test Progress"=0, "Test Progress Text"=""} ("Progress")) -> ()
        n182 = Index Array(array=w289, index=w288) -> (element=w287:string)
        n183 = call <vilib>:"NT Write String.vi"("String"=w287, "Name"="TestMode/TestName") -> ()  [unwired: 9 in, 1 out]
        n184 = property on="Progress" class="Clust (strict)"("Visible"=TRUE) -> ()  [unwired: 2 in, 2 out]
        n185 = property on="Motor" class="Clust (strict)"("Visible"=w284) -> ()  [unwired: 2 in, 2 out]
        n186 = property on="Test Slider" class="Slide (strict)"("Visible"=w284) -> ()  [unwired: 2 in, 2 out]
        n187 = property on="On/Off" class="Bool (strict)"("Visible"=w284) -> ()  [unwired: 2 in, 2 out]
        n188 = property on="Rev/Fwd" class="Clust (strict)"("Visible"=w284) -> ()  [unwired: 2 in, 2 out]
        n189 = property on="Test Ring" class="Ring (strict)"("Visible"=w284) -> ()  [unwired: 2 in, 2 out]
      }
      event "Listbox": Double Click {
        # "Shift clears all"
        # "Update symbols on the listbox"
        n190 = event-data() -> ("PlatMods.Shift"=w292:bool, "Row"=w294:i32)  [unwired: 1 in]
        n191 = case shown="True" w292 {
          tunnel: w294 -> [w298 _]
          tunnel: 1 -> [w297 _]
          frame False {
            n192 = property on="Listbox" class="LstBox (strict)"() -> ("Item Symbols"=w296:i32[])  [unwired: 2 in, 2 out]
            n193 = Replace Array Subset(array=w296, new element=w297, index=w298) -> (w295:i32[])
            n194 = property on="Listbox" class="LstBox (strict)"("Item Symbols"=w295) -> ()  [unwired: 2 in, 2 out]
          }
          frame True {
            w299 = 0 ("Top Row")
            n195 = property on="Listbox" class="LstBox (strict)"() -> ("Number of Rows"=w301:u32)  [unwired: 2 in, 2 out]
            n196 = Initialize Array(0, w301) -> (w300:i32[])
            n197 = property on="Listbox" class="LstBox (strict)"("Top Row"=w299, "Value"=w299, "Item Symbols"=w300) -> ()  [unwired: 2 in, 2 out]
          }
        }
      }
      event "Listbox": Key Down {
        # "Update symbols on the listbox\nLeft and right keys check and uncheck"
        n198 = event-data() -> ("VKey"=w305:T20)  [unwired: 1 in]
        n199 = case shown="\"Left\", \"Right\"" w305 {
          selector: w305 -> [w310 _]
          tunnel: eventvkey."Left" ("VKey") -> [w308 _]
          frame "Left", "Right" {
            n200 = Equal?(x=w308, y=w310) -> (x = y?=w309:bool)
            n201 = Select(t=0, s=w309, f=1) -> (s? t:f=w311:i32)
            n202 = property on="Listbox" class="LstBox (strict)"() -> ("Item Symbols"=w314:i32[])  [unwired: 2 in, 2 out]
            n203 = Replace Array Subset(array=w314, new element=w311, index="Listbox") -> (w313:i32[])
            n204 = property on="Listbox" class="LstBox (strict)"("Item Symbols"=w313) -> ()  [unwired: 2 in, 2 out]
          }
          frame Default {
          }
        }
      }
      event "DB Camera Config": Value Change {
        # "Show or hide the cluster of controls, store in ini file"
        n205 = event-data() -> ("NewVal"=w318:bool)  [unwired: 1 in]
        n206 = case shown="False" w318 {
          tunnel: w317 -> [w327 _]
          tunnel: [w320 w338] -> w316
          tunnel: w315 -> [w319 w338]
          frame False {
            w334 = "Camera"
            w337 = FALSE ("Visible")
            n207 = local read "Camera Settings"() -> (w326:T3)
            n208 = Index Array(array=w327) -> (element=w330:cluster{string[]})  [unwired: 1 in]
            n209 = Unbundle(w326) -> ("Frame Rate"=w325:i32, "Compression"=w324:i32, "Size"=w328:u16)
            n210 = Unbundle(w330) -> (w329:string[])
            n211 = Index Array(array=w329, index=w328) -> (element=w323:string)
            n212 = call-poly <vilib>:"Write Key.vi"("section"=w334, "value"=w323, "key"="Size", "refnum"=w319) -> ("refnum out"=w336:T18)  [unwired: 2 in, 5 out]
            n213 = call-poly <vilib>:"Write Key.vi"("section"=w334, "value"=w325, "key"="FrameRate", "refnum"=w336) -> ("refnum out"=w335:T18)  [unwired: 1 in, 6 out]
            n214 = property on="Camera Settings" class="Clust (strict)"("Visible"=w337) -> ()  [unwired: 2 in, 2 out]
            n215 = local write "DB Camera Config"(w337) -> ()
            n216 = call-poly <vilib>:"Write Key.vi"("section"=w334, "value"=w324, "key"="Compression", "refnum"=w335) -> ("refnum out"=w321:T18)  [unwired: 1 in, 6 out]
            n217 = call <vilib>:"Close Config Data.vi"("refnum"=w321) -> ("file path"=w322:path)  [unwired: 2 in, 8 out]
            n218 = call <vilib>:"Open Config Data.vi"("configuration file path"=w322) -> ("refnum"=w320:T18)  [unwired: 8 in, 2 out]
          }
          frame True {
            n219 = property on="Camera Settings" class="Clust (strict)"("Visible"=TRUE) -> ()  [unwired: 2 in, 2 out]
          }
        }
      }
      event "Camera Settings": Value Change {
        # "Update summary string when any elements of DB camera change"
        n220 = event-data() -> ("NewVal"=w351:T3)  [unwired: 1 in]
        n221 = Index Array(array=w347) -> (element=w346:cluster{string[]})  [unwired: 1 in]
        n222 = Unbundle(w351) -> ("Frame Rate"=w342:i32, "Compression"=w341:i32, "Size"=w344:u16)
        n223 = Unbundle(w346) -> (w345:string[])
        n224 = Index Array(array=w345, index=w344) -> (element=w343:string)
        n225 = Format Into String(format string="%s   %dfps   %d%%", w343, w342, w341) -> (resulting string=w348:string)  [unwired: 2 in, 1 out]
        n226 = Build Array(w348) -> (w349:string[])
        n227 = property on="DB Camera Config" class="Bool (strict)"("Strings [4]"=w349) -> ()  [unwired: 2 in, 2 out]
      }
      event "Motor.Enable": Value Change {
        # "When the test mode otor enable helper is set, update that\ntree row item's value"
        n228 = event-data() -> ("NewVal"=w357:bool)  [unwired: 1 in]
        n229 = Unbundle("Motor") -> ("Value"=w356:dbl)  [unwired: 1 out]
        n230 = Select(t=w356, s=w357, f=0.0) -> (s? t:f=w354:dbl)
        n231 = call <vilib>:"NT Write Number.vi"("Numeric"=w354, "Name"=w353) -> ()  [unwired: 9 in, 1 out]
      }
      event "Test Slider": Value Change {
        # "When the test mode slider helper is set, update that\ntree row item's value"
        n232 = event-data() -> ("NewVal"=w360:dbl)  [unwired: 1 in]
        n233 = call <vilib>:"NT Write Number.vi"("Numeric"=w360, "Name"=w361) -> ()  [unwired: 9 in, 1 out]
      }
      event "On/Off": Value Change {
        # "When the test mode on/off helper value is set, update that\ntree row item's value"
        n234 = event-data() -> ("NewVal"=w365:bool)  [unwired: 1 in]
        n235 = Boolean To (0,1)(Boolean=w365) -> (0, 1=w364:i16)
        n236 = call <vilib>:"NT Write Number.vi"("Numeric"=w364, "Name"=w363) -> ()  [unwired: 9 in, 1 out]
      }
      event "Rev/Fwd": Value Change {
        # "When the test mode helper value for relays is set, update that\ntree row item's value"
        n237 = event-data() -> ("NewVal.Forward"=w373:bool, "NewVal.Reverse"=w372:bool)  [unwired: 1 in]
        n238 = Boolean To (0,1)(Boolean=w373) -> (0, 1=w369:i16)
        n239 = Boolean To (0,1)(Boolean=w372) -> (0, 1=w371:i16)
        n240 = Negate(x=w371) -> (-x=w370:i16)
        n241 = Add(x=w369, y=w370) -> (x+y=w368:i16)
        n242 = call <vilib>:"NT Write Number.vi"("Numeric"=w368, "Name"=w367) -> ()  [unwired: 9 in, 1 out]
      }
      event "Test Ring": Value Change {
        # "When a test mode helper value is selected from the ring,\nset the tree item's variable to the string value"
        n243 = event-data() -> ("NewVal"=w377:u16)  [unwired: 1 in]
        n244 = property on="Test Ring" class="Ring (strict)"() -> ("Strings []"=w378:string[])  [unwired: 2 in, 2 out]
        n245 = Index Array(array=w378, index=w377) -> (element=w376:string)
        n246 = call <vilib>:"NT Write String.vi"("String"=w376, "Name"=w375) -> ()  [unwired: 9 in, 1 out]
      }
      event "Rec Mode": Value Change {
        # "Update globals for recording mode and path to read log from.\nClear when logging and let NetworkTables set path for vision to\nuse."
        n247 = event-data() -> ("NewVal"=w388:enum32{"Stop", "Record", "Playback"})  [unwired: 1 in]
        n248 = global write "WPI_DashboardLogging Global.vi" "Logging Filename"(path "") -> ()
        n249 = case shown="\"Playback\"" w388 {
          tunnel: w387 -> [_ w390 w398]
          tunnel: [_ _ w397] -> w384
          tunnel: [_ _ w396] -> _
          tunnel: w382 -> [_ _ w394]
          tunnel: cluster{i32, i32} {-250, 170} -> [_ _ w393]
          tunnel: [_ _ T21 {"Image Size"=TRUE, "Image Type"=TRUE, "Pixel Value"=TRUE, "ROI Information"=TRUE, "Zoom Factor"=FALSE} ("Image Information Shown:All Elements")] -> w380
          tunnel: [_ _ TRUE ("Zoom Factor")] -> w379
          frame Default {
          }
          frame "Stop", "Record" {
            # "Place Window too"
            n250 = invoke class="VI" method="FP.Close"(reference=w390) -> (reference out=w389:refnum<vi>)  [unwired: 2 in, 2 out]
            n251 = invoke class="VI" method="Abort VI"(reference=w389) -> ()  [unwired: 2 in, 3 out]
          }
          frame "Playback" {
            n252 = call "Open Playback Panel.vi"("Offset"=w393, "DB VI Ref"=w394, "Playback in"=w398) -> ("Playback out"=w395:refnum<vi>)  [unwired: 8 in]
            n253 = register-events(w395) -> (reference out=w397:refnum<event-registration>, error out=w396:errorcluster)  [unwired: 2 in]
          }
        }
        n254 = global write "WPI_DashboardLogging Global.vi" "Recording"(w388) -> ()
        n255 = property on="Camera Image" class="ImageControl"("Image Information Shown"=w380, "Image Information Visible"=w379) -> ()  [unwired: 2 in, 2 out]
        n256 = call <vilib>:"WPI_DashboardNT Log FieldName Cache.vi"("Operation"=enum16{"Lookup/Add", "Index", "Clear"}."Clear") -> ()  [unwired: 8 in, 3 out]
      }
      event Panel Close {
        w399 = enum32{"Stop", "Record", "Playback"}."Stop" ("Rec Mode")
        # "Playback window has been closed, abort"
        n257 = event-data() -> ()  [unwired: 1 in, 4 out]
        n258 = local write "Rec Mode"(w399) -> ()
        n259 = global write "WPI_DashboardLogging Global.vi" "Recording"(w399) -> ()
      }
      event Panel Close {
        # "Abort playback window and ourself"
        n260 = event-data() -> ()  [unwired: 1 in, 4 out]
        n261 = invoke class="VI" method="FP.Close"(reference=w404) -> (reference out=w403:refnum<vi>)  [unwired: 2 in, 2 out]
        n262 = invoke class="VI" method="Abort VI"(reference=w403) -> (error out=w402:errorcluster)  [unwired: 2 in, 2 out]
        n263 = invoke class="VI" method="Abort VI"(error in=w402) -> ()  [unwired: 2 in, 3 out]
      }
      event "Vision": Value Change {
        # "Enable/Disable Compression slider.\nHW USB is hard-coded into the camera"
        n264 = event-data() -> ("NewVal"=w410:u16)  [unwired: 1 in]
        n265 = Equal?(x=w410, y=u32 2 ("milliseconds to wait")) -> (x = y?=w408:bool)
        n266 = Select(t=T22."Disabled and Grayed Out" ("Disabled"), s=w408, f=T22."Enabled" ("Disabled")) -> (s? t:f=w405:T22)
        n267 = property on="Compression" class="Slide (strict)"("DisabledEnum"=w405) -> ()  [unwired: 2 in, 2 out]
      }
    }
  }
  n268 = while {
    tunnel: w38 -> [w413]
    i -> [w416]
    stop <- FALSE stop-if-true
    n269 = Wait (ms)(milliseconds to wait=u32 100) -> ()  [unwired: 1 out]
    n270 = case shown="\"Playback\"" "Rec Mode" {
      tunnel: w416 -> [_ _ w431]
      tunnel: [u32 2829099 ("Base Color") u32 11141120 ("Target Color") w420] -> w412
      frame "Stop", Default {
        # "Reset the color, extra updates don't cost much"
      }
      frame "Record" {
      }
      frame "Playback" {
        # "Playback"
        n271 = Quotient & Remainder(x=w431, y=u32 50 ("milliseconds to wait")) -> (x-y*floor(x/y)=w427:u32)  [unwired: 1 out]
        n272 = Divide(x=w427, y=u32 50 ("milliseconds to wait")) -> (x/y=w424:dbl)
        n273 = Multiply(x=6.283185307179586, y=w424) -> (x*y=w429:dbl)
        n274 = Sine(x=w429) -> (sin(x)=w428:dbl)
        n275 = Absolute Value(x=w428) -> (abs(x)=w421:dbl)
        n276 = call "Interpolate RGB Color.vi"("Proportion"=w421, "Target Color"=u32 30976, "Base Color"=u32 2829099) -> ("Result Color"=w420:u32)  [unwired: 8 in]
      }
    }
    n277 = property class="Pane"(reference=w413, "PaneColor"=w412) -> ()  [unwired: 1 in, 2 out]
  }
  n278 = TCP Create Listener(10:u16 1741 ("timeout ms (25000)")) -> (3:w1:refnum<k5>)  [unwired: 4 in, 2 out]
  n279 = while {
    tunnel: w1 -> [w433]
    stop <- FALSE stop-if-true
    n280 = TCP Wait On Listener(11:w433) -> (4:w432:refnum<k5>)  [unwired: 3 in, 4 out]
    n281 = local write "TCP"(w432) -> ()
  }
  n282 = property on="On/Off" class="Bool (strict)"("Visible"=w6) -> ()  [unwired: 2 in, 2 out]
  n283 = property on="Motor" class="Clust (strict)"("Visible"=w6) -> ()  [unwired: 2 in, 2 out]
  n284 = property on="Progress" class="Clust (strict)"("Visible"=w6) -> ()  [unwired: 2 in, 2 out]
  n285 = property on="Test Ring" class="Ring (strict)"("Visible"=w6) -> ()  [unwired: 2 in, 2 out]
  n286 = property on="Rev/Fwd" class="Clust (strict)"("Visible"=w6) -> ()  [unwired: 2 in, 2 out]
  n287 = property on="Camera Settings" class="Clust (strict)"("Visible"=w6) -> ()  [unwired: 2 in, 2 out]
  n288 = local write "DB Camera Config"(w6) -> ()
  n289 = global write "WPI_DashboardLogging Global.vi" "Recording"(w32) -> ()
  n290 = local write "Rec Mode"(w32) -> ()
